vi "NewTicker.vi"(11 "Period":u32) -> (3 "Ticker":refnum<class "Ticker.lvclass">)   [LabVIEW 2013, in "Ticker.lvclass"]
uses:
  Ticker.lvclass
  Ticker.lvclass/Ticker.ctl
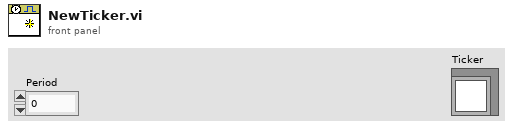
[diagram p1: front panel]
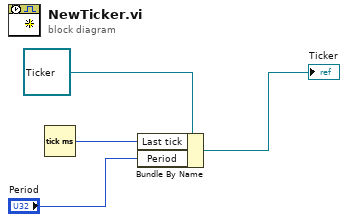
[diagram p0: block diagram]
diagram:
  n1 = Tick Count (ms)() -> (millisecond timer value=w3:u32)
  n2 = Bundle By Name(cluster=refnum<class "Ticker.lvclass"> refnum ("Ticker"), "Last tick"=w3, "Period"="Period") -> (→"Ticker":refnum<class "Ticker.lvclass">)
